vi "get_calibration.vi"(8 "error in (no error)":errorcluster, 11 "GenericTrajectory.lvclass in":refnum<class "TrajectoryDL091126GenericVoxel.lvclass">) -> (0 "error out":errorcluster, 2 "calibration":T1, 3 "GenericTrajectory.lvclass out":refnum<class "TrajectoryDL091126GenericVoxel.lvclass">)   [LabVIEW 2010, in "TrajectoryDL091126GenericVoxel.lvclass"]
uses:
  TrajectoryDL091126GenericVoxel.lvclass
  common/clusters/calibration.ctl
  common/enumerations/unit.ctl
  TrajectoryDL091126GenericVoxel.lvclass/TrajectoryDL091126GenericVoxel.ctl
  common/classes/Image/Image/Image.lvclass
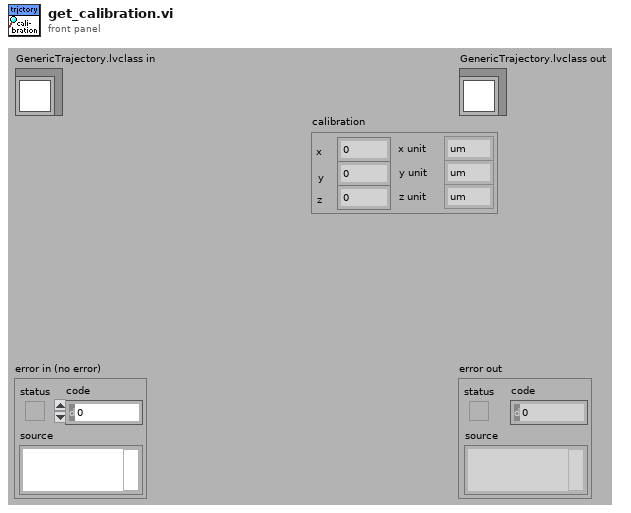
[diagram p1: front panel]
types:
  T1 = typedef "calibration.ctl" = cluster{"x":dbl, "y":dbl, "z":dbl, "x unit":T2, "y unit":T2, "z unit":T2}
  T2 = typedef "Image.lvclass/unit.ctl" = enum16{"um", "s"}
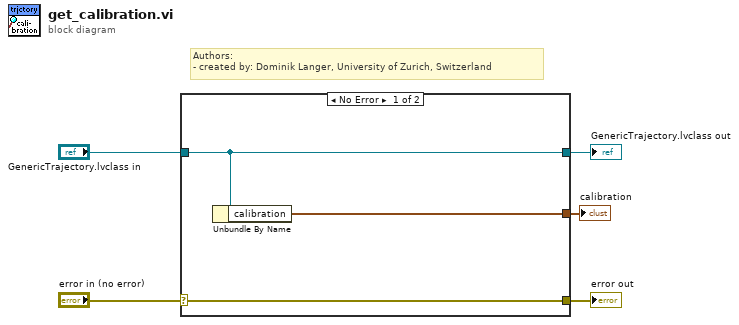
[diagram p0: block diagram]
diagram:
  # "Authors: \n- created by: Dominik Langer, University of Zurich, Switzerland"
  n1 = case shown="No Error" "error in (no error)" {
    selector: "error in (no error)" -> [w8 w9]
    tunnel: [w8 w9] -> w4
    tunnel: [w7 w10] -> w2
    tunnel: "GenericTrajectory.lvclass in" -> [w7 w10]
    tunnel: [w6 _] -> w1
    frame No Error {
      n2 = Unbundle By Name(w7) -> ("calibration"=w6:T1)
    }
    frame Error {
    }
  }
  "error out" <- w4
  "GenericTrajectory.lvclass out" <- w2
  "calibration" <- w1
